vi "RouteGuide RouteChat Read.vi"(7 "Occurrence":enum16{"With Occurrence", "Without Occurrence"}(ring), 8 "error in":errorcluster, 11 "Call ID in":T3) -> (0 "error out":errorcluster, 1 "Success":bool, 2 "Response Data":T1, 3 "Call ID":T3)   [LabVIEW 2019, in "route_guide_client.lvlib"]
uses:
  route_guide_client.lvlib
  <vilib>/gRPC/LabVIEW gRPC Library/Shared/grpcId.ctl
  RPC Messages/routeguide_RouteNote.ctl
  RPC Messages/routeguide_Point.ctl
  RPC Messages/routeguide_RouteNote_Flat.ctl
  RPC Messages/routeguide_Point_Flat.ctl
  aea5dbbb-03a2-479b-ad95-94da4ee1cea9.vi
  <vilib>/gRPC/LabVIEW gRPC Library/Shared/TranslateGrpcError.vi
  <vilib>/gRPC/LabVIEW gRPC Library/Shared/Wait On Occurence.vi
  RPC Messages/FlatToRichrouteguide_Point.vi
  <vilib>/gRPC/LabVIEW gRPC Library/Server API/Server/Get Server DLL Path.vi
  <vilib>/Utility/error.llb/Error Cluster From Error Code.vi
  <vilib>/gRPC/LabVIEW gRPC Library/grpc-lvsupport-release.lvlib
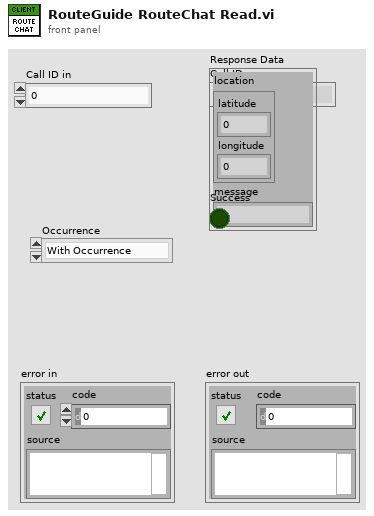
[diagram p1: front panel]
types:
  T1 = typedef "route_guide_client.lvlib/routeguide_RouteNote.ctl" = cluster{"location":T2, "message":string}
  T2 = typedef "route_guide_client.lvlib/routeguide_Point.ctl" = cluster{"latitude":i32, "longitude":i32}
  T3 = typedef "grpc-lvsupport-release.lvlib/grpcId.ctl" = u64
  T4 = typedef "route_guide_client.lvlib/routeguide_RouteNote_Flat.ctl" = cluster{"location":T5, "message":string}
  T5 = typedef "route_guide_client.lvlib/routeguide_Point_Flat.ctl" = cluster{"latitude":i32, "longitude":i32}
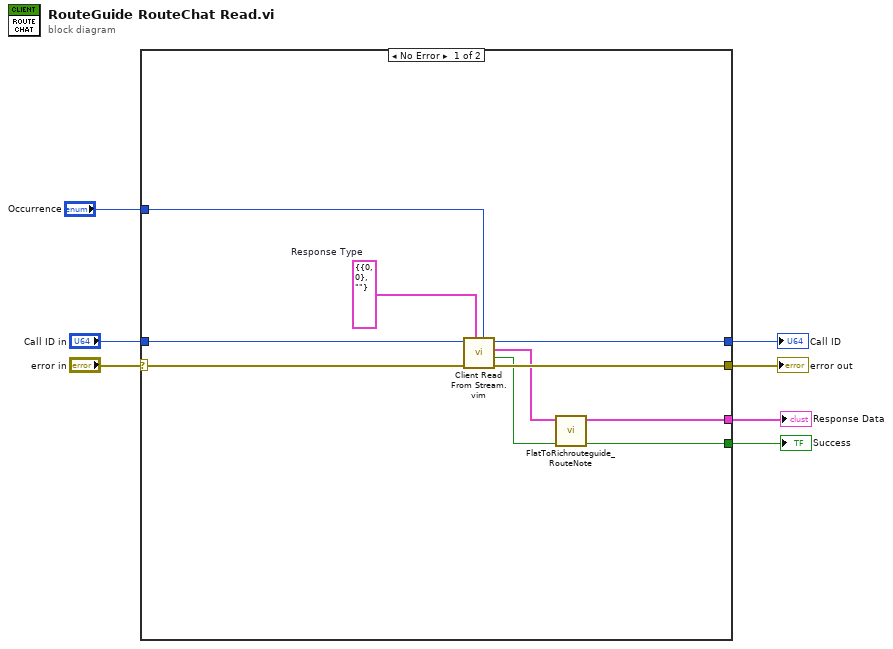
[diagram p0: block diagram]
diagram:
  n1 = case shown="No Error" "error in" {
    selector: "error in" -> [w16 w17]
    tunnel: [w15 w17] -> w6
    tunnel: "Call ID in" -> [w14 w18]
    tunnel: [w12 w18] -> w4
    tunnel: [w9 _] -> w3
    tunnel: [w13 _] -> w2
    tunnel: "Occurrence" -> [w8 _]
    frame No Error {
      w11 = T4 {"location"={"latitude"=0, "longitude"=0}, "message"=""}  # Response Type
      n2 = call "Client Read From Stream.vim"("Occurrence"=w8, "Response Type"=w11, "error in"=w16, "Call ID in"=w14) -> ("error out"=w15:errorcluster, "Success"=w13:bool, "Response Data"=w10:T4, "Call ID out"=w12:u64)  [unwired: 4 in]
      n3 = call "FlatToRichrouteguide_RouteNote.vi"("InputCluster"=w10) -> ("OutputCluster"=w9:T1)  [unwired: 10 in]
    }
    frame Error {
    }
  }
  "error out" <- w6
  "Call ID" <- w4
  "Response Data" <- w3
  "Success" <- w2
